vi "create server acceptor.vi"(8 "error in":errorcluster, 9 "port":u16, 11 "engine pointer":u64) -> (0 "error out":errorcluster, 3 "server acceptor out":refnum<class "server acceptor.lvclass">)   [LabVIEW 2016, in "server acceptor.lvclass"]
uses:
  server acceptor.lvclass
  C:/Users/IEUser/Desktop/libasynclvtls/tls classes/connection creator/connection creator.lvclass
  dllwrapper/tls new socket user event.ctl
  server acceptor.lvclass/server acceptor.ctl
  dllwrapper/library path.vi
  connection creator.lvclass
  dllwrapper/async tls dl.lvlib
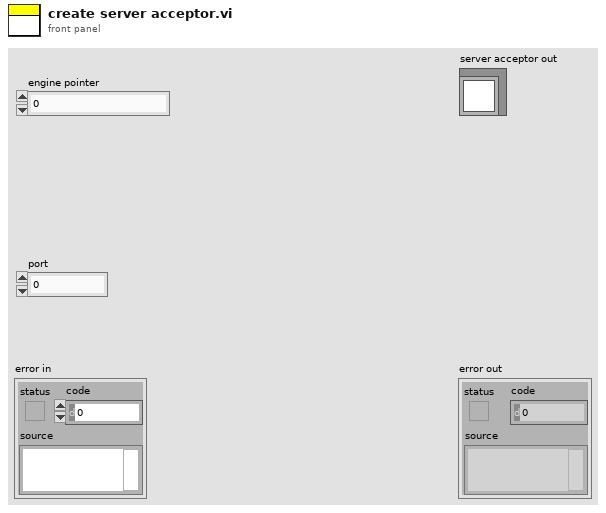
[diagram p1: front panel]
types:
  T1 = typedef "async tls dl.lvlib/tls new socket user event.ctl" = cluster{"request type":u32, "request ID":u32, "error code":i32, "errstring":string, "connection":u64}
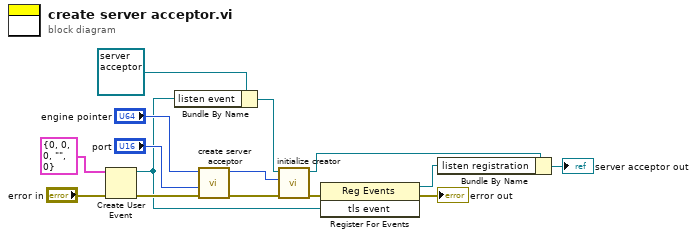
[diagram p0: block diagram]
diagram:
  n1 = Create User Event(user event datatype=T1 {"request type"=0, "request ID"=0, "error code"=0, "errstring"="", "connection"=0} ("tls event"), error in="error in") -> (user event=w3:refnum<user-event>, error out=w7:errorcluster)
  n2 = Bundle By Name(cluster=refnum<class "server acceptor.lvclass"> refnum ("client connector.lvclass"), "listen event"=w3) -> (w6:refnum<class "server acceptor.lvclass">)
  n3 = call "create server acceptor.vi"("error in"=w7, "port"="port", "engine"="engine pointer") -> ("error out"=w15:errorcluster, "acceptor out"=w10:u64)  [unwired: 7 in]
  n4 = call "initialize creator.vi"("error in"=w15, "pointer"=w10, "connection creator in"=w6) -> ("error out"=w14:errorcluster, "connection creator out"=w9:refnum<class "server acceptor.lvclass">)  [unwired: 7 in]
  n5 = register-events(error in=w14, w3) -> (reference out=w1:refnum<event-registration>, error out=→"error out":errorcluster)  [unwired: 1 in]
  n6 = Bundle By Name(cluster=w9, "listen registration"=w1) -> (→"server acceptor out":refnum<class "server acceptor.lvclass">)
